vi "wait for 335(SubVI).vi"(8 "delay":dbl format="%#_13g", 11 "队列输出":refnum<queue>) -> ()   [LabVIEW 2019, in "SubVI.lvlib"]
uses:
  SubVI.lvlib
  config.ctl
  Instrument.ctl
  lib/QDInstrument.dll
  <vilib>/NI/Modbus Library/API/Master/Modbus Master.lvclass
panel:
  # "(真是通道1，假是通道2)"
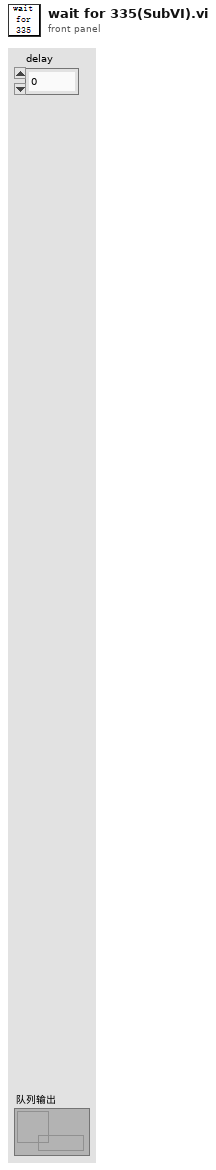
[diagram p1: front panel]
types:
  T1 = typedef "config.ctl" = cluster{"initialize":string, "6221":cluster{"6221 Resource":refnum<visa-resource-name>, "Delta status":bool}, "7001":cluster{"Ch":bool}, "SR830+6221":cluster{"source":u16, "阻抗":dbl, "量程入 4":i32, "量程入 3":i32, "量程入 2":i32, "量程入 1":i32, "电流":dbl, "SR830 2":bool, "SR830 3":bool, "SR830 4":bool, "SR830 1":bool, "VISA 1":refnum<visa-resource-name>, "VISA 2":refnum<visa-resource-name>, "VISA 3":refnum<visa-resource-name>, "VISA 4":refnum<visa-resource-name>, "量程":enum16{"量程每次测量会判定", "量程不变为设定值"}}, "2400":cluster{"2400":bool, "VISA":refnum<visa-resource-name>}, "ch":cluster{"ch str":string, "ch1":bool, "ch2":bool, "布尔":bool}, "error":bool, "数据文件路径":path, "log":cluster{"log路径":path, "log interval":dbl}, "Instrument":T2}
  T2 = typedef "Instrument.ctl" = cluster{"335 Resource":refnum<visa-resource-name>, "Input (0:A)":u16, "Instrument Type":i32, "quantum design":refnum<k24>, "Heater Output (1:1)":u16, "335state":refnum<vi>, "semaphore":T3, "TCP master instance":refnum<class "Modbus Master.lvclass">}
  T3 = typedef "Semaphore RefNum" = refnum<k1>
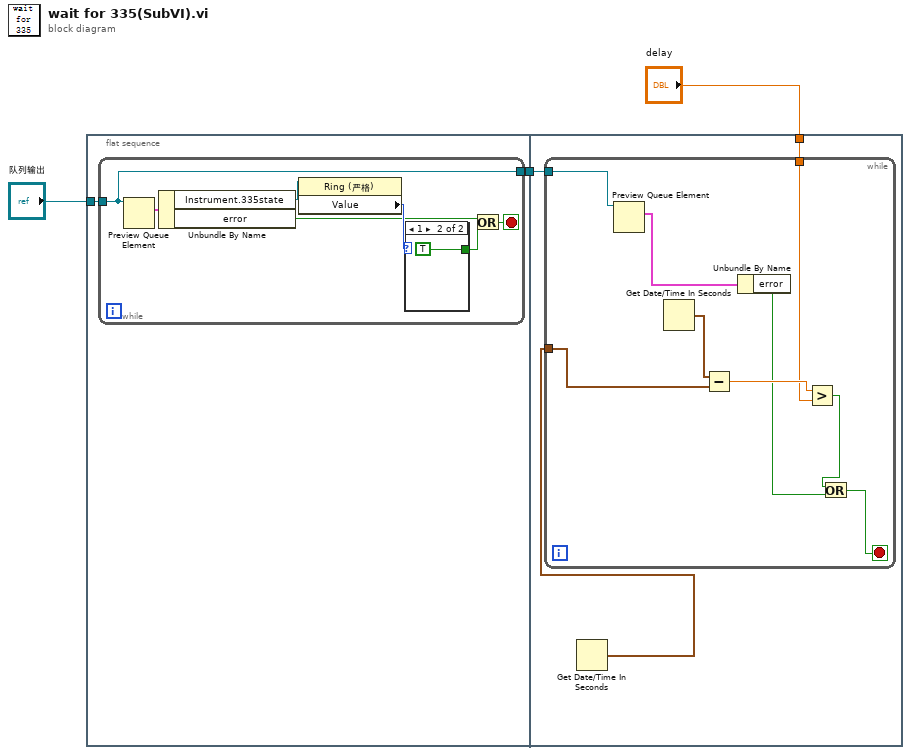
[diagram p0: block diagram]
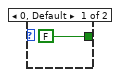
[diagram p2: hidden frame]
diagram:
  n1 = flat-sequence {
    tunnel: "队列输出" -> [w5]
    tunnel: [w4] -> w1
    tunnel: "delay" -> [w16]
    tunnel: w1 -> [w15]
    frame #0 {
      n2 = while {
        tunnel: w5 -> [w6]
        tunnel: [w6] -> w4
        stop <- w12 stop-if-true
        n3 = Preview Queue Element(queue=w6) -> (element=w7:T1)  [unwired: 2 in, 3 out]
        n4 = Unbundle By Name(w7) -> ("Instrument.335state"=w10:refnum<vi>, "error"=w8:bool)
        n5 = property class="Ring (严格)"(reference=w10) -> ("Value"=w9:i32)  [unwired: 1 in, 2 out]
        n6 = case shown="1" w9 {
          tunnel: [FALSE TRUE] -> w11
          frame 0, Default {
          }
          frame 1 {
          }
        }
        n7 = Or(x=w8, y=w11) -> (x .or. y?=w12:bool)
      }
    }
    frame #1 {
      n8 = Get Date/Time In Seconds() -> (seconds since 1Jan1904=w17:timestamp)
      n9 = while {
        tunnel: w17 -> [w25]
        tunnel: w16 -> [w23]
        tunnel: w15 -> [w22]
        stop <- w18 stop-if-true
        n10 = Preview Queue Element(queue=w22) -> (element=w21:T1)  [unwired: 2 in, 3 out]
        n11 = Get Date/Time In Seconds() -> (seconds since 1Jan1904=w26:timestamp)
        n12 = Subtract(x=w26, y=w25) -> (x-y=w24:dbl)
        n13 = Unbundle By Name(w21) -> ("error"=w19:bool)
        n14 = Greater?(x=w24, y=w23) -> (0:w20:bool)
        n15 = Or(x=w20, y=w19) -> (x .or. y?=w18:bool)
      }
    }
  }
